vi "WriteAO.vi"(8 "error in (no error)":errorcluster, 9 "Array":dbl[](array[numeric]), 10 "Analog Output":T1, 11 "VISA resource name":refnum<visa-resource-name>) -> (0 "error out":errorcluster, 3 "VISA resource name out":refnum<visa-resource-name>)   [LabVIEW 2020, in "HandsOnPi2040.lvlib"]
doc: "Establishes communication with the instrument and optionally performs an instrument identification query and/or an instrument reset. It also places the instrument in a default state needed for other instrument driver operations. Therefore, call this VI before calling other instrument driver VIs for this instrument. Generally, you need to call the <b>Initialize</b> VI only once at the beginning of an application."
uses:
  <instrlib>/HandsOnPi2040/HandsOnPi2040.lvlib
  <instrlib>/HandsOnPi2040/Public/AOs.ctl
panel:
  # "Input"
  # "Output"
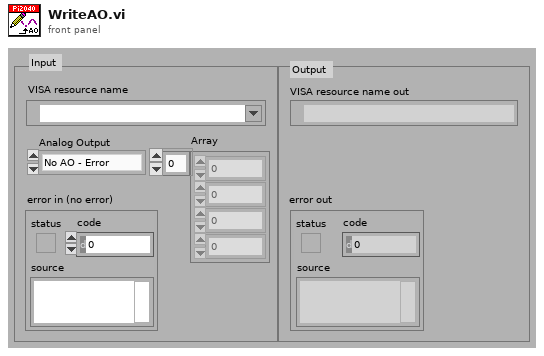
[diagram p1: front panel]
types:
  T1 = typedef "HandsOnPi2040.lvlib/AOs.ctl" = enum16{"No AO - Error", "AO1"}
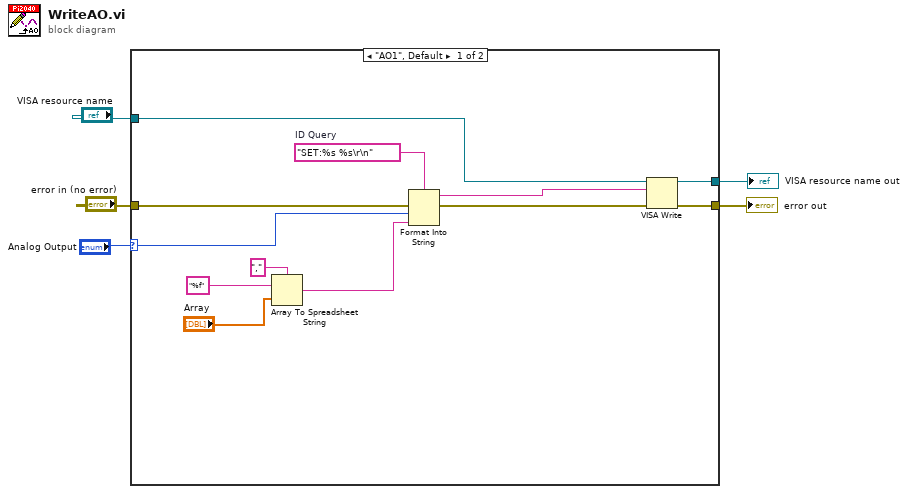
[diagram p0: block diagram]
diagram:
  n1 = case shown="\"AO1\", Default" "Analog Output" {
    selector: "Analog Output" -> [w17 _]
    tunnel: [w13 w19] -> w2
    tunnel: [w12 w18] -> w3
    tunnel: "VISA resource name" -> [w11 w18]
    tunnel: "error in (no error)" -> [w10 w19]
    frame "AO1", Default {
      w16 = "SET:%s %s\r\n"  # ID Query
      n2 = Array To Spreadsheet String(delimiter (Tab)=",", array="Array", 3:"%f" ("format string")) -> (spreadsheet string=w7:string)
      n3 = Format Into String(format string=w16, error in=w10, w17, w7) -> (resulting string=w15:string, error out=w14:errorcluster)  [unwired: 1 in]
      n4 = VISA Write(VISA resource name=w11, write buffer=w15, error in (no error)=w14) -> (VISA resource name out=w12:refnum<visa-resource-name>, error out=w13:errorcluster)  [unwired: 1 out]
    }
    frame "No AO - Error" {
    }
  }
  "VISA resource name out" <- w3
  "error out" <- w2
